vi "EmergencyStopAll.vi"() -> ()   [LabVIEW 2022 SP3]
uses:
  DriveConfigGlobal.vi
  GenericDriveCommand.ctl
  Anemometry/Anemometry Sub Vis/Globals/Trav_pos_global.vi
  Anemometry/Anemometry Sub Vis/Gen Trav/Route mapping/Route_mapping_global.vi
panel:
  out "Traverse Name":string
  out "Position Offset":sgl[](array[numeric]) format="%.2f"
  out "Tunnel Coordinates":sgl[](array[numeric]) format="%.2f"
  in  "stop":bool
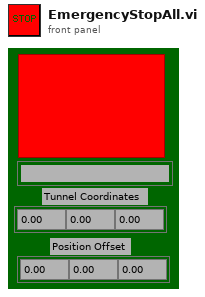
[diagram p1: front panel]
types:
  T1 = enum32{"Invalid", "Default", "Floating", "Floating/Auto-Hide", "Modal"}
  T2 = typedef "GenericDriveCommand.ctl" = string
  T3 = typedef "DriveProperties.ctl" = cluster{"Channel Name":string, "Vel. Default":sgl, "Acc. Default":sgl, "Vel. Max":sgl, "Vel. Min":sgl, "Acc. Max":sgl, "Acc. Min":sgl, "Pulses/unit":sgl, "Address":u8, "Pulse Offset":i32, "Pos Tolerance":sgl, "Pulses/rev":sgl, "Backlash/Eng units":sgl, "Current Pos":sgl, "Ch Status":enum16{"Active", "Offline", "Simulate"}, "Port Name":string, "Axis Transform mode":string, "Metadata Ch Name":string, "Type":T4, "De Power Motor":enum16{"TRUE", "FALSE"}, "ConfigString":string}
  T4 = typedef "Traverse Type.ctl" = enum16{"MCode", "Dynamixel"}
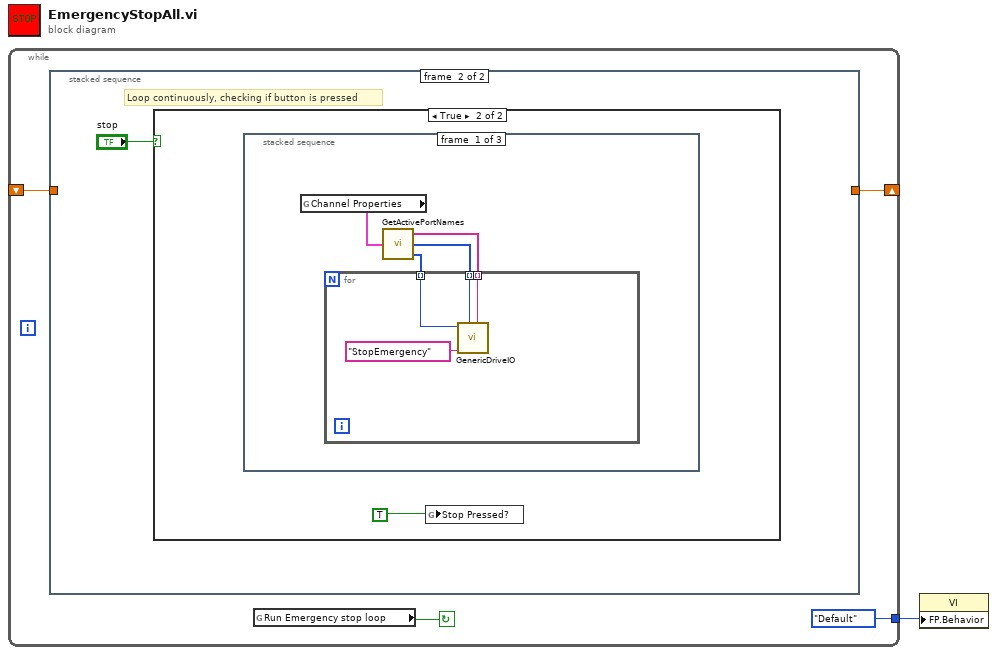
[diagram p0: block diagram]
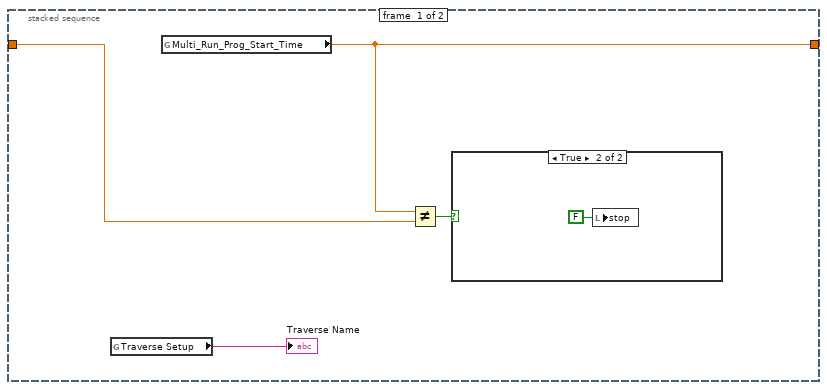
[diagram p2: hidden frame]
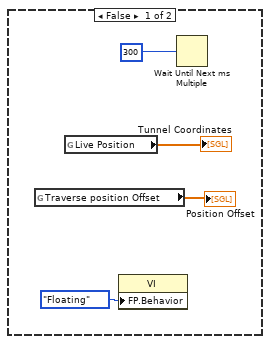
[diagram p4: hidden frame]
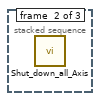
[diagram p5: hidden frame]
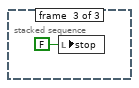
[diagram p6: hidden frame]
diagram:
  n1 = while {
    shift-right: [w4] -> _
    shift-left: _ -> [w3]
    tunnel: [T1."Default" ("Front Panel Window:Behavior")] -> w1
    stop <- w5 continue-if-true
    n2 = stacked-sequence {
      tunnel: [w9 _] -> w4
      tunnel: w3 -> [w8 _]
      frame #0 {
        n3 = global read "Route_mapping_global.vi" "Traverse Setup"() -> (→"Traverse Name":string)
        n4 = global read "Trav_pos_global.vi" "Multi_Run_Prog_Start_Time"() -> (w9:dbl)
        n5 = Not Equal?(x=w9, y=w8) -> (x != y?=w7:bool)
        n6 = case shown="True" w7 {
          frame False {
          }
          frame True {
            n7 = local write "stop"(FALSE ("stop")) -> ()
          }
        }
      }
      frame #1 {
        # "Loop continuously, checking if button is pressed"
        n8 = case shown="True" "stop" {
          frame False {
            n9 = global read "Trav_pos_global.vi" "Traverse position Offset"() -> (→"Position Offset":sgl[])
            n10 = global read "Trav_pos_global.vi" "Live Position"() -> (→"Tunnel Coordinates":sgl[])
            n11 = property class="VI"("FP.Behavior"=T1."Floating" ("Front Panel Window:Behavior")) -> ()  [unwired: 2 in, 2 out]
            n12 = Wait Until Next ms Multiple(millisecond multiple=u32 300) -> ()  [unwired: 1 out]
          }
          frame True {
            n13 = stacked-sequence {
              frame #0 {
                n14 = global read "DriveConfigGlobal.vi" "Channel Properties"() -> (w20:T3[])
                n15 = call "GetActivePortNames.vi"("Channel Properties"=w20) -> ("Port Name Array"=w19:string[], "Drive Type Array"=w18:T4[], "Address"=w17:u8[])
                n16 = for {
                  tunnel: w19 -> [w24] mode=indexing
                  tunnel: w18 -> [w22] mode=indexing
                  tunnel: w17 -> [w21] mode=indexing
                  n17 = call "GenericDriveIO.vi"("GenericDriveCommand"=T2 "StopEmergency", "Address"=w21, "Type"=w22, "Port Name"=w24) -> ()  [unwired: 5 in, 3 out]
                }
              }
              frame #1 {
                n18 = call "Shut_down_all_Axis.vi"() -> ()  [unwired: 1 in, 1 out]
              }
              frame #2 {
                n19 = local write "stop"(FALSE ("stop")) -> ()
              }
            }
            n20 = global write "DriveConfigGlobal.vi" "Stop Pressed?"(TRUE) -> ()
          }
        }
      }
    }
    n21 = global read "DriveConfigGlobal.vi" "Run Emergency stop loop"() -> (w5:bool)
  }
  n22 = property class="VI"("FP.Behavior"=w1) -> ()  [unwired: 2 in, 2 out]
